vi "Copy.vi"(8 "Error In":errorcluster, 11 "Tree Data":refnum<class "Tree Data.lvclass">) -> (0 "Error Out":errorcluster, 2 "Copy":refnum<class "Tree Data.lvclass">)   [LabVIEW 2020, in "NI_VIAnCFGDataStructure.lvlib" / "Tree Data.lvclass"]
doc: "This is a base method defining an interface for Tree Data Copy functionality, invoked in the Tree API with Copy methods. Override it in child classes. The default copy implementation is LV fork."
uses:
  <vilib>/addons/analyzer/VIAnCFGDataStructure/Tree Data/Tree Data.lvclass
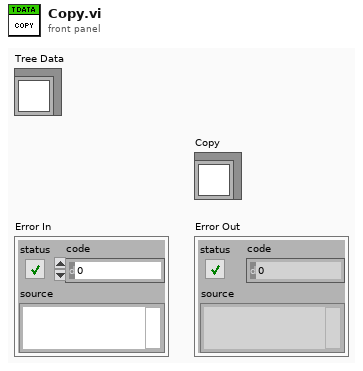
[diagram p1: front panel]
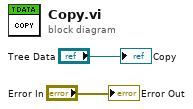
[diagram p0: block diagram]
diagram:
  "Copy" <- "Tree Data"
  "Error Out" <- "Error In"
